vi "Save meas device config.vi"(7 "Equipo a Utilizar":enum16{"SR830 Lock In", "TDS 2012B Osciloscope"}(ring), 8 "error in (no error)":errorcluster, 9 "Datos Osciloscopio":T2 {"Número Promedio" min=2 max=20}, 10 "Datos Lock In":T1, 11 "Refnum in":T3) -> (0 "error out":errorcluster, 3 "Refnum out":T3)   [LabVIEW 2020]
uses:
  <vilib>/Utility/config.llb/NI_LVConfig.lvlib
  <vilib>/Utility/config.llb/Write Key (String).vi
  <vilib>/Utility/config.llb/Write Key (I32).vi
  <vilib>/Utility/config.llb/Config Data RefNum.ctl
  Type Definitions/datos osciloscopio.ctl
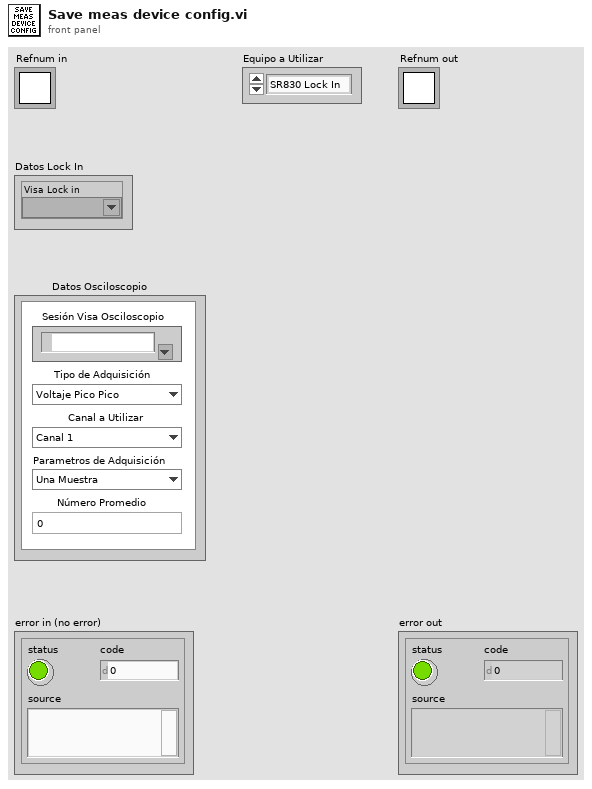
[diagram p1: front panel]
types:
  T1 = cluster{"Visa Lock in":refnum<visa-resource-name>}
  T2 = typedef "datos osciloscopio.ctl" = cluster{"Sesión Visa Osciloscopio":refnum<visa-resource-name>, "Tipo de Adquisición":enum16{"Voltaje Pico Pico", "Voltaje RMS", "Cursor Tiempo"}, "Canal a Utilizar":enum16{"Canal 1", "Canal 2", "Canal 1 y 2"}, "Parametros de Adquisición":enum16{"Una Muestra", "Promedio"}, "Número Promedio":i32}
  T3 = typedef "NI_LVConfig.lvlib/Config Data RefNum.ctl" = refnum<k1>
  T4 = enum16{"Voltaje Pico Pico", "Voltaje RMS", "Cursor Tiempo"}
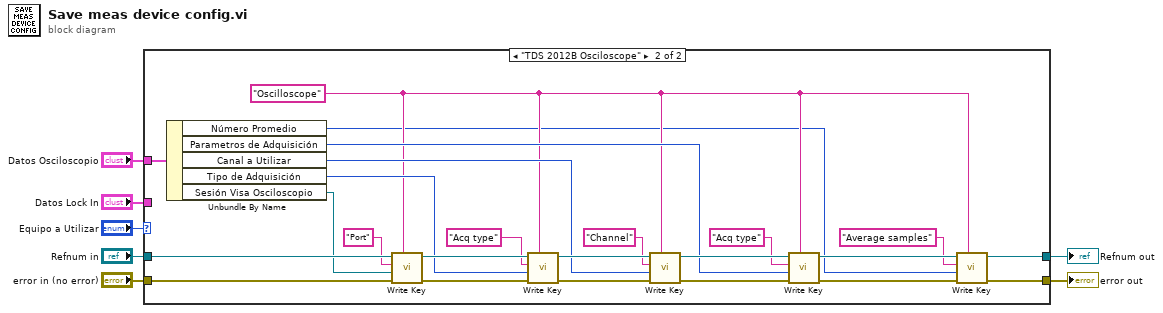
[diagram p0: block diagram]
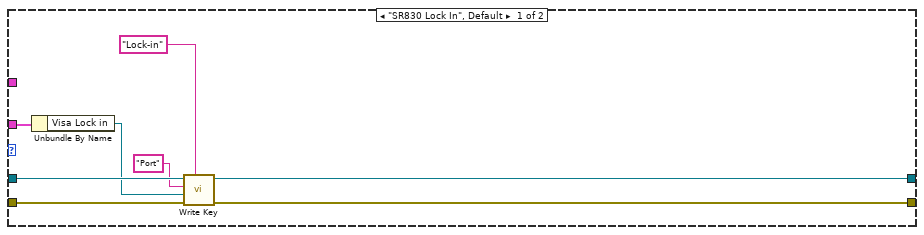
[diagram p2: hidden frame]
diagram:
  n1 = case shown="\"TDS 2012B Osciloscope\"" "Equipo a Utilizar" {
    tunnel: "error in (no error)" -> [w15 w39]
    tunnel: [w14 w21] -> w3
    tunnel: "Datos Lock In" -> [w11 _]
    tunnel: "Datos Osciloscopio" -> [_ w36]
    tunnel: "Refnum in" -> [w13 w37]
    tunnel: [w12 w19] -> w7
    frame "SR830 Lock In", Default {
      n2 = Unbundle By Name(w11) -> ("Visa Lock in"=w8:refnum<visa-resource-name>)
      n3 = call-poly <vilib>:"Write Key.vi"("section"="Lock-in", "error in (no error)"=w15, "value"=w8, "key"="Port", "refnum"=w13) -> ("error out"=w14:errorcluster, "refnum out"=w12:T3)  [unwired: 4 in, 1 out]
    }
    frame "TDS 2012B Osciloscope" {
      w18 = "Oscilloscope" ("section")
      n4 = Unbundle By Name(w36) -> ("Número Promedio"=w17:i32, "Parametros de Adquisición"=w22:enum16{"Una Muestra", "Promedio"}, "Canal a Utilizar"=w26:enum16{"Canal 1", "Canal 2", "Canal 1 y 2"}, "Tipo de Adquisición"=w30:T4, "Sesión Visa Osciloscopio"=w35:refnum<visa-resource-name>)
      n5 = call-poly <vilib>:"Write Key.vi"("section"=w18, "error in (no error)"=w39, "value"=w35, "key"="Port", "refnum"=w37) -> ("error out"=w38:errorcluster, "refnum out"=w32:T3)  [unwired: 4 in, 1 out]
      n6 = call-poly <vilib>:"Write Key.vi"("section"=w18, "error in (no error)"=w38, "value"=w30, "key"="Acq type", "refnum"=w32) -> ("error out"=w33:errorcluster, "refnum out"=w28:T3)  [unwired: 4 in, 1 out]
      n7 = call-poly <vilib>:"Write Key.vi"("section"=w18, "error in (no error)"=w33, "value"=w26, "key"="Channel", "refnum"=w28) -> ("error out"=w29:errorcluster, "refnum out"=w24:T3)  [unwired: 4 in, 1 out]
      n8 = call-poly <vilib>:"Write Key.vi"("section"=w18, "error in (no error)"=w29, "value"=w22, "key"="Acq type", "refnum"=w24) -> ("error out"=w25:errorcluster, "refnum out"=w20:T3)  [unwired: 4 in, 1 out]
      n9 = call-poly <vilib>:"Write Key.vi"("section"=w18, "error in (no error)"=w25, "value"=w17, "key"="Average samples", "refnum"=w20) -> ("error out"=w21:errorcluster, "refnum out"=w19:T3)  [unwired: 4 in, 1 out]
    }
  }
  "Refnum out" <- w7
  "error out" <- w3
